vi "Rename Script.vi"   [LabVIEW 2021]
uses:
  <vilib>/Utility/EditLVLibs/Edit LVLibs.lvlib
  <vilib>/Utility/EditLVProj/Edit LVProj.lvlib
types:
  T1 = typedef "Edit LVProj.lvlib/Library And VI References.ctl" = cluster{"Target Reference":refnum<vi>, "VI References":refnum<vi>[], "Library References":refnum<vi>[]}
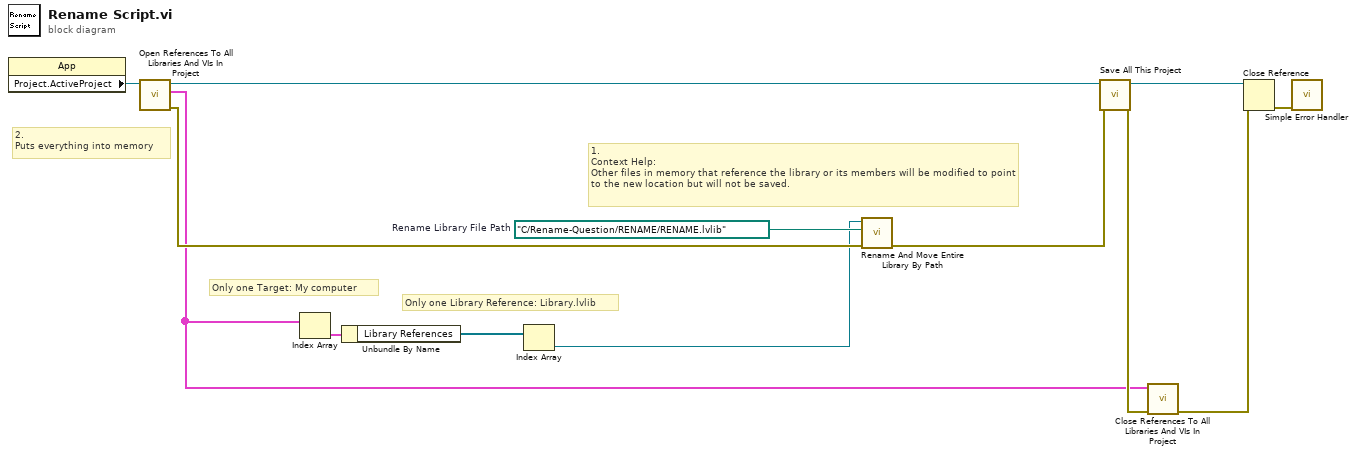
[diagram p0: block diagram]
diagram:
  w9 = path "C:/Rename-Question/RENAME/RENAME.lvlib"  # Rename Library File Path
  # "Only one Library Reference: Library.lvlib"
  # "Only one Target: My computer"
  # "2.\nPuts everything into memory"
  # "1.\nContext Help:\nOther files in memory that reference the library or its members will be modified to point to the new location but will not be saved."
  n1 = property class="App"() -> ("Project.ActiveProject"=w13:refnum<vi>)  [unwired: 2 in, 2 out]
  n2 = call <vilib>:"Open References To All Libraries And VIs In Project.vi"("Project in"=w13) -> ("error out"=w4:errorcluster, "VI and Library References"=w1:T1[], "Project out"=w5:refnum<vi>)  [unwired: 8 in]
  n3 = Index Array(array=w1) -> (element=w6:T1)  [unwired: 1 in]
  n4 = Unbundle By Name(w6) -> ("Library References"=w3:refnum<vi>[])
  n5 = Index Array(array=w3) -> (element=w2:refnum<vi>)  [unwired: 1 in]
  n6 = call <vilib>:"Rename And Move Entire Library By Path.vi"("error in (no error)"=w4, "New library path"=w9, "Library ref in"=w2) -> ("error out"=w7:errorcluster)  [unwired: 7 in, 1 out]
  n7 = call <vilib>:"Save All This Project.vi"("error in (no error)"=w7, "Project in"=w5) -> ("error out"=w11:errorcluster, "Project out"=w12:refnum<vi>)  [unwired: 8 in]
  n8 = call <vilib>:"Close References To All Libraries And VIs In Project.vi"("error in (no error)"=w11, "VI and Library References"=w1) -> ("error out"=w10:errorcluster)  [unwired: 9 in]
  n9 = Close Reference(reference=w12, error in (no error)=w10) -> (error out=w8:errorcluster)
  n10 = call <vilib>:"Simple Error Handler.vi"("error in (no error)"=w8) -> ()  [unwired: 4 in, 5 out]
